vi "trigger.vi"(6 "US/sham trig":u32, 7 "initial string":string, 8 "enable":bool, 9 "Eye tracker":u32, 10 "EEG":u32, 11 "VISA resource name":refnum<visa-resource-name>) -> (3 "success":bool)   [LabVIEW 2019]
panel:
  out "receive from trig box":string="set delay ack\n"
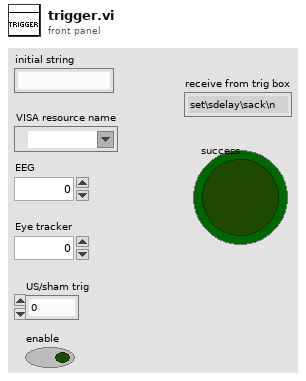
[diagram p1: front panel]
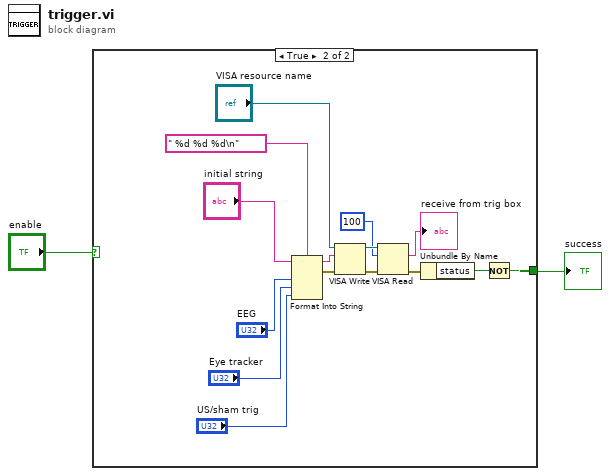
[diagram p0: block diagram]
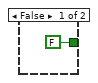
[diagram p2: hidden frame]
diagram:
  n1 = case shown="True" "enable" {
    tunnel: [FALSE w7] -> w2
    frame False {
    }
    frame True {
      n2 = Format Into String(format string=" %d %d %d\n", initial string="initial string", "EEG", "Eye tracker", "US/sham trig") -> (resulting string=w16:string, error out=w5:errorcluster)  [unwired: 1 in]
      n3 = VISA Write(VISA resource name="VISA resource name", write buffer=w16, error in (no error)=w5) -> (VISA resource name out=w15:refnum<visa-resource-name>, error out=w4:errorcluster)  [unwired: 1 out]
      n4 = VISA Read(VISA resource name=w15, byte count=u32 100, error in (no error)=w4) -> (read buffer=→"receive from trig box":string, error out=w6:errorcluster)  [unwired: 2 out]
      n5 = Unbundle By Name(w6) -> ("status"=w11:bool)
      n6 = Not(x=w11) -> (.not. x?=w7:bool)
    }
  }
  "success" <- w2
